vi "Global 1.vi"() -> ()   [LabVIEW 2023]
panel:
  out "SERVO_OUTPUT_RAW":T1
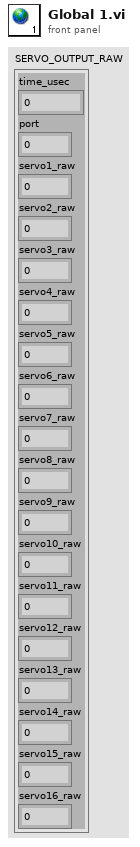
[diagram p1: front panel]
types:
  T1 = cluster{"time_usec":u32, "port":u8, "servo1_raw":u16, "servo2_raw":u16, "servo3_raw":u16, "servo4_raw":u16, "servo5_raw":u16, "servo6_raw":u16, "servo7_raw":u16, "servo8_raw":u16, "servo9_raw":u16, "servo10_raw":u16, "servo11_raw":u16, "servo12_raw":u16, "servo13_raw":u16, "servo14_raw":u16, "servo15_raw":u16, "servo16_raw":u16}
diagram:
